vi "Gen Stage 4 Update Supporting Projects.vi"(7 "Staus":refnum<vi>, 8 "error in (no error)":errorcluster, 10 "New Name":string, 11 "Template Project Path":path) -> (0 "error out":errorcluster)   [LabVIEW 2021, in "Plugin Generator.lvlib"]
uses:
  Plugin Generator.lvlib
  <vilib>/CIF Foundation/CIF LabVIEW Scripting/LV Scripting/LV Scripting Utilities.lvlib
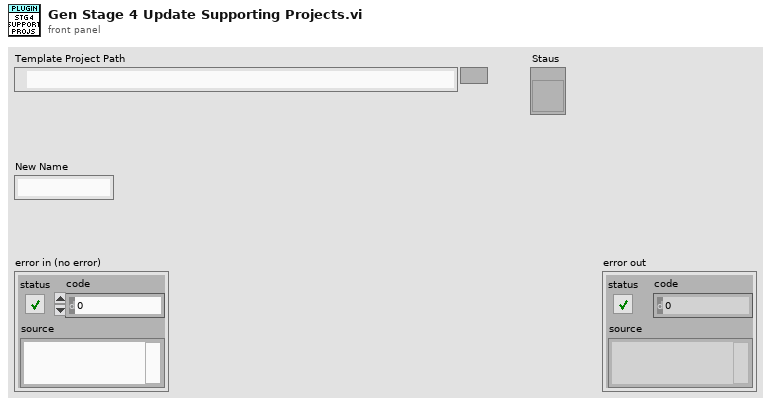
[diagram p1: front panel]
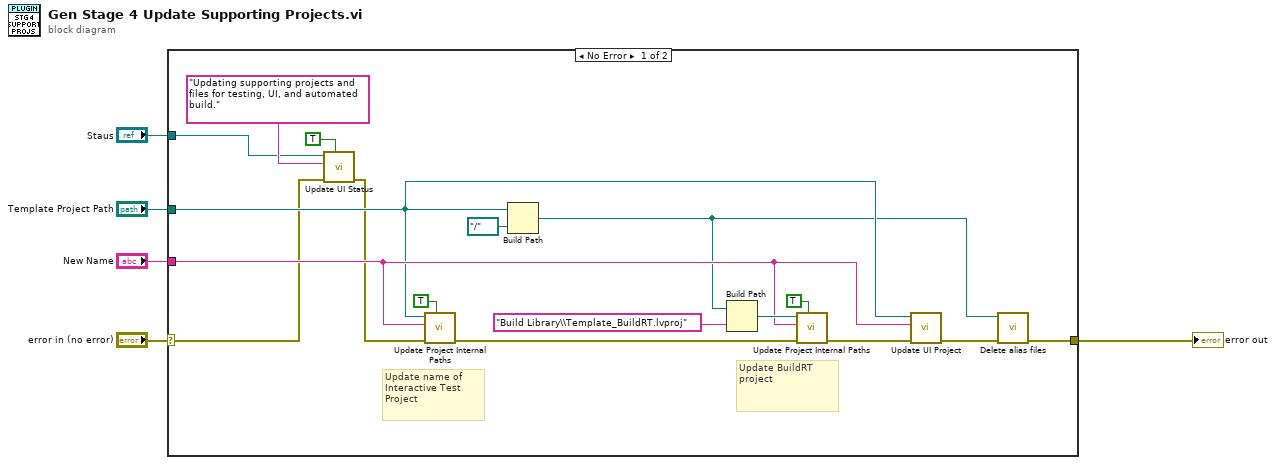
[diagram p0: block diagram]
diagram:
  n1 = case shown="No Error" "error in (no error)" {
    selector: "error in (no error)" -> [w10 w23]
    tunnel: "New Name" -> [w16 _]
    tunnel: "Template Project Path" -> [w15 _]
    tunnel: [w7 w23] -> w3
    tunnel: "Staus" -> [w12 _]
    frame No Error {
      # "Update BuildRT project"
      # "Update name of Interactive Test Project"
      n2 = call "Update UI Status.vi"("Previous Complete"=TRUE, "error in"=w10, "Status to Display"="Updating supporting projects and files for testing, UI, and automated build." ("To display"), "String in"=w12) -> ("error out"=w11:errorcluster)  [unwired: 7 in]
      n3 = call <vilib>:"Update Project Internal Paths.vi"("Rename Project"=TRUE, "error in (no error)"=w11, "New Subname"=w16, "Project Path"=w15) -> ("error out"=w14:errorcluster)  [unwired: 7 in]
      n4 = Build Path(base path=w15, name or relative path=path "../..") -> (appended path=w6:path)
      n5 = Build Path(base path=w6, name or relative path="Build Library\\Template_BuildRT.lvproj" ("Class Name")) -> (appended path=w20:path)
      n6 = call <vilib>:"Update Project Internal Paths.vi"("Rename Project"=TRUE, "error in (no error)"=w14, "New Subname"=w16, "Project Path"=w20) -> ("error out"=w17:errorcluster)  [unwired: 7 in]
      n7 = call "Update UI Project.vi"("error in (no error)"=w17, "New Name"=w16, "Template Project Path"=w15) -> ("error out"=w8:errorcluster)  [unwired: 8 in]
      n8 = call "Delete alias files.vi"("error in"=w8, "Directory Path"=w6) -> ("error out"=w7:errorcluster)  [unwired: 9 in]
    }
    frame Error {
    }
  }
  "error out" <- w3
